vi "FPGA-Trap-Test.vi"() -> ()   [LabVIEW 2010]
uses:
  <vilib>/eio/EIONode/EIONode.xnode
  <vilib>/rvi/eio/nirviEIOImplementation/nirviEIOImplementation.xnode
  <vilib>/rvi/eio/common/nirviEmuClasses.ctl
  <vilib>/rvi/eio/common/nirviEmuTemplateMethod_noerrors.vi
panel:
  out "AIWidrTrap2":fxp<+/-,26,5> format="%.23g"
  in  "5VTrap2":bool
  in  "stop":bool
  out "AIWidrTrap1":fxp<+/-,26,5> format="%.23g"
  in  "5VTrap1":bool
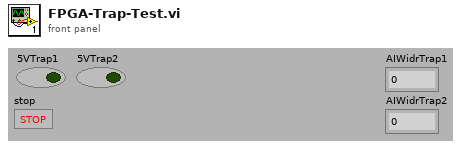
[diagram p1: front panel]
types:
  T1 = typedef "nirviEmuClasses.ctl" = enum16{"IO Read", "IO Write", "Method", "Property Read", "Property Write"}
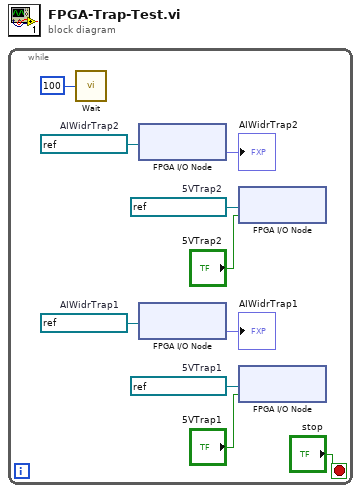
[diagram p0: block diagram]
diagram:
  n1 = while {
    stop <- "stop" stop-if-true
    w2 = refnum<k21> "Mod1/AI31"  # AIWidrTrap2
    w4 = refnum<k21> "Mod6/DIO20"  # 5VTrap2
    w7 = refnum<k21> "Mod1/AI30"  # AIWidrTrap1
    w10 = refnum<k21> "Mod6/DIO21"  # 5VTrap1
    n2 = call "Wait"("Count(mSec)"=u32 100) -> ()  [unwired: 1 out]
    n3 = xnode "FPGA I/O Node"("FPGA I/O In"=w2) -> ("I/O Item"=→"AIWidrTrap2":fxp<+/-,26,5>)  [unwired: 1 out]
    n4 = xnode "FPGA I/O Node"("FPGA I/O In"=w7) -> ("I/O Item"=→"AIWidrTrap1":fxp<+/-,26,5>)  [unwired: 1 out]
    n5 = xnode "FPGA I/O Node"("I/O Item"="5VTrap2", "FPGA I/O In"=w4) -> ()  [unwired: 1 out]
    n6 = xnode "FPGA I/O Node"("I/O Item"="5VTrap1", "FPGA I/O In"=w10) -> ()  [unwired: 1 out]
  }
